vi "TCP_SenData.vi"(1 "Server":T1 {"Knob" scale=0.0..10.0; "Horizontal Fill Slide" scale=0.0..10.0}, 8 "error in":errorcluster, 11 "Clients":refnum<k5>[](array[refnum])) -> (0 "error out":errorcluster, 2 "# of Connections":i32, 3 "Clients":refnum<k5>[](array[refnum]), 5 "Current Data":dbl)   [LabVIEW 2020, in "TCP_Server.lvlib"]
uses:
  TCP_Server.lvlib
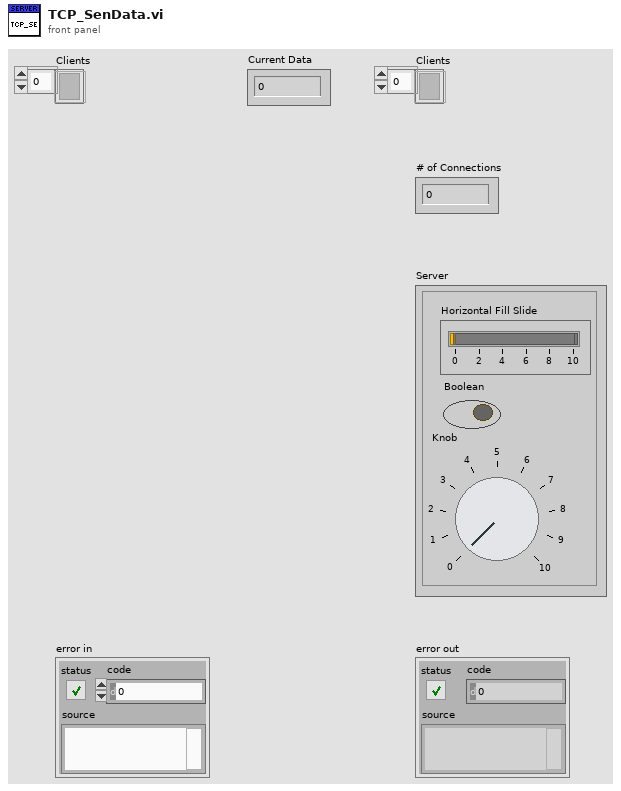
[diagram p1: front panel]
types:
  T1 = cluster{"Horizontal Fill Slide":dbl, "Knob":dbl, "Boolean":bool}
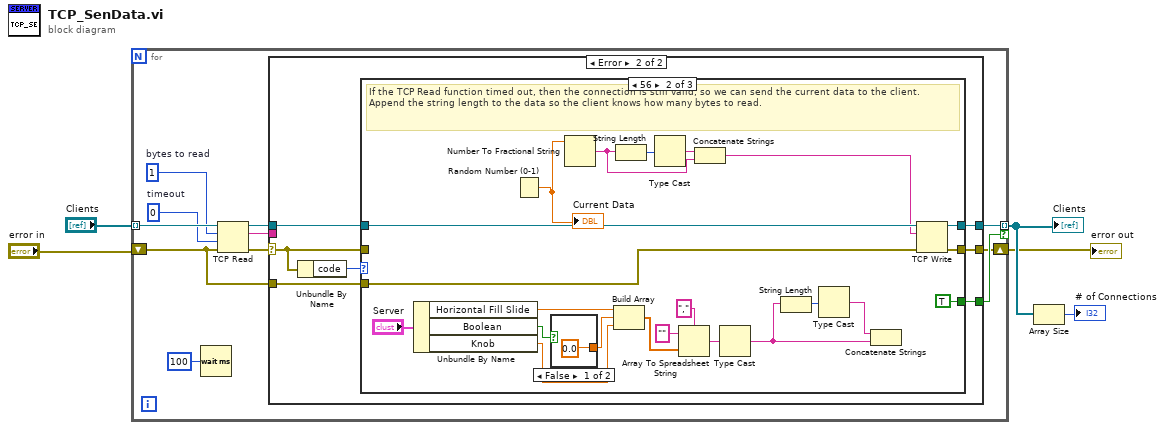
[diagram p0: block diagram]
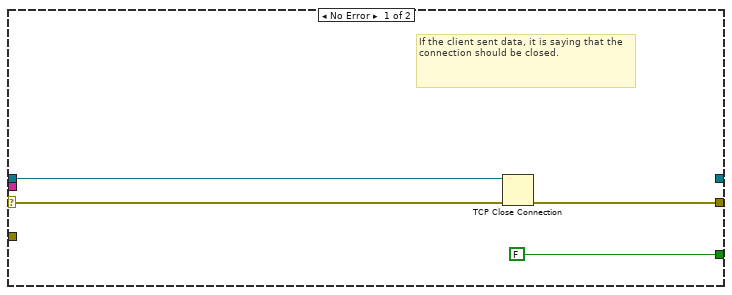
[diagram p2: hidden frame]
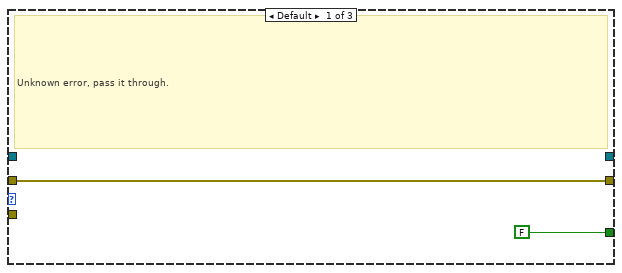
[diagram p3: hidden frame]
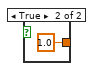
[diagram p4: hidden frame]
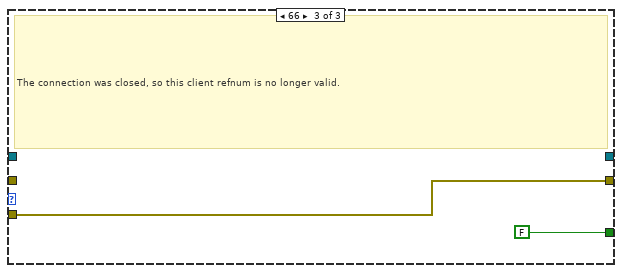
[diagram p5: hidden frame]
diagram:
  n1 = for {
    tunnel: "Clients" -> [w16] mode=indexing
    shift-right: [w8] -> w1
    shift-left: "error in" -> [w7]
    tunnel: [w10] -> w4 mode=indexing if=w9
    w13 = 0  # timeout
    w14 = 1  # bytes to read
    n2 = Wait (ms)(milliseconds to wait=u32 100) -> ()  [unwired: 1 out]
    n3 = TCP Read(connection ID=w16, bytes to read=w14, error in (no error)=w7, 9:w13) -> (connection ID out=w15:refnum<k5>, data out=w11:string, error out=w12:errorcluster)  [unwired: 1 out]
    n4 = case shown="Error" w12 {
      selector: w12 -> [w19 w26]
      tunnel: w15 -> [w20 w23]
      tunnel: w11 -> [_ _]
      tunnel: [_ w21] -> w10
      tunnel: [FALSE w22] -> w9
      tunnel: [w17 w25] -> w8
      tunnel: w7 -> [_ w24]
      frame No Error {
        # "If the client sent data, it is saying that the connection should be closed."
        # "If the client sent data, it is saying that the connection should be closed."
        n5 = TCP Close Connection(connection ID=w20, error in (no error)=w19) -> (error out=w17:errorcluster)  [unwired: 2 out]
      }
      frame Error {
        # "Ignore connection closed and timeout errors"
        n6 = Unbundle By Name(w26) -> ("code"=w27:i32)
        n7 = case shown="56" w27 {
          tunnel: w26 -> [w29 _ _]
          tunnel: [w29 w51 w55] -> w25
          tunnel: w24 -> [_ w47 w55]
          tunnel: w23 -> [_ w50 _]
          tunnel: [FALSE TRUE FALSE] -> w22
          tunnel: [_ w49 _] -> w21
          frame Default {
            # "Unknown error, pass it through."
          }
          frame 56 {
            # "If the TCP Read function timed out, then the connection is still valid, so we can send the current data to the client. Append the string length to the data so the client knows how many bytes to read."
            n8 = Unbundle By Name("Server") -> ("Horizontal Fill Slide"=w39:dbl, "Boolean"=w45:bool, "Knob"=w43:dbl)
            n9 = Random Number (0-1)() -> (number: 0 to 1=w31:dbl)
            "Current Data" <- w31
            n10 = case shown="False" w45 {
              tunnel: [0.0 1.0] -> w46
              frame False {
              }
              frame True {
              }
            }
            n11 = Number To Fractional String(number=w31) -> (F-format string=w32:string)  [unwired: 3 in]
            n12 = Build Array(w39, w46, w43) -> (w44:dbl[])
            n13 = String Length(string=w32) -> (length=w33:i32)
            n14 = Type Cast(x=w33) -> (*(type *) &x=w34:string)  [unwired: 1 in]
            n15 = Array To Spreadsheet String(delimiter (Tab)=",", array=w44, 3:"" ("format string")) -> (spreadsheet string=w35:string)
            n16 = Concatenate Strings(w34, w32) -> (w30:string)
            n17 = Type Cast(x=w35) -> (*(type *) &x=w36:string)  [unwired: 1 out]
            n18 = String Length(string=w36) -> (length=w42:i32)
            n19 = Type Cast(x=w42) -> (*(type *) &x=w37:string)  [unwired: 1 out]
            n20 = Concatenate Strings(w37, w36) -> ()  [unwired: 1 out]
            n21 = TCP Write(connection ID=w50, data in=w30, error in (no error)=w47) -> (connection ID out=w49:refnum<k5>, error out=w51:errorcluster)  [unwired: 2 out]
          }
          frame 66 {
            # "The connection was closed, so this client refnum is no longer valid."
          }
        }
      }
    }
  }
  "Clients" <- w4
  "error out" <- w1
  n22 = Array Size(array=w4) -> (size(s)=→"# of Connections":i32)
